vi "_Config Updated.vi"(8 "error in (no error)":errorcluster, 10 "Config Map":map{string, string}(c390), 11 "VisaResource in":refnum<class "VisaResource.lvclass">) -> (0 "error out":errorcluster, 3 "VisaResource out":refnum<class "VisaResource.lvclass">)   [LabVIEW 2020, in "PicoG-Core.lvlib" / "VisaResource.lvclass"]
uses:
  VisaResource.lvclass
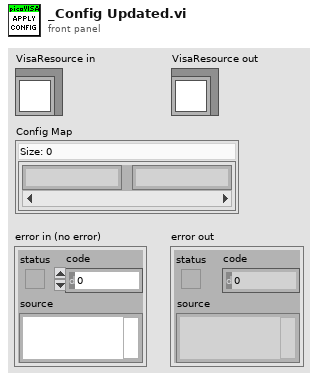
[diagram p1: front panel]
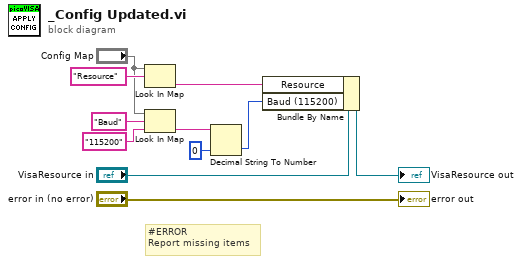
[diagram p0: block diagram]
diagram:
  # "#ERROR\nReport missing items"
  n1 = Look In Map(map="Config Map", key="Resource") -> (value=w7:string)  [unwired: 1 in, 1 out]
  n2 = Look In Map(map="Config Map", key="Baud", default value="115200" ("key")) -> (value=w3:string)  [unwired: 1 out]
  n3 = Decimal String To Number(string=w3, default (0L)=u32 0 ("default (0 I32)")) -> (number=w2:u32)  [unwired: 1 in, 1 out]
  n4 = Bundle By Name(cluster="VisaResource in", "Resource"=w7, "Baud (115200)"=w2) -> (→"VisaResource out":refnum<class "VisaResource.lvclass">)
  "error out" <- "error in (no error)"
